vi "Create FIFO FGV Queues.vi"(8 "error in (no error)":errorcluster) -> (0 "error out":errorcluster, 4 "BC FIFO Idx Qs":T1)   [LabVIEW 2011, in "AIT 1553 Custom Device.lvlib"]
uses:
  AIT 1553 Custom Device.lvlib
  RT Controls/FIFO Idx Qs.ctl
panel:
  out "FIFO Idx Qs":T1
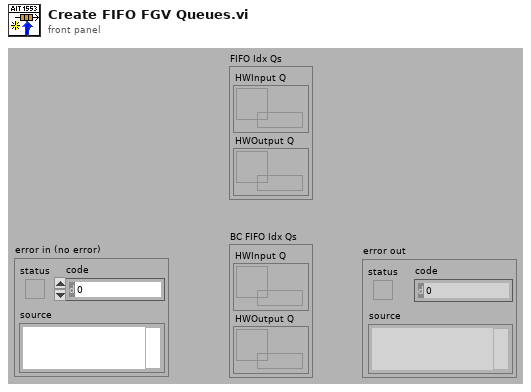
[diagram p1: front panel]
types:
  T1 = typedef "AIT 1553 Custom Device.lvlib/FIFO Idx Qs.ctl" = cluster{"HWInput Q":refnum<queue>, "HWOutput Q":refnum<queue>}
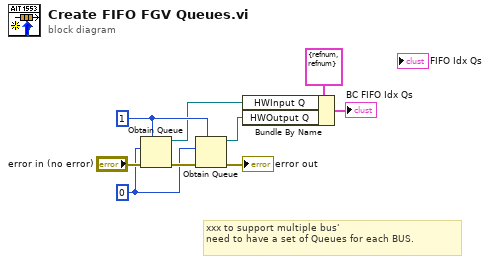
[diagram p0: block diagram]
diagram:
  w5 = 1 ("max queue size (-1, unlimited)")
  w6 = 0
  # "xxx to support multiple bus'\nneed to have a set of Queues for each BUS."
  n1 = Obtain Queue(max queue size (-1, unlimited)=w5, element data type=w6, error in (no error)="error in (no error)") -> (queue out=w3:refnum<queue>, error out=w8:errorcluster)  [unwired: 2 in, 1 out]
  n2 = Obtain Queue(max queue size (-1, unlimited)=w5, element data type=w6, error in (no error)=w8) -> (queue out=w2:refnum<queue>, error out=→"error out":errorcluster)  [unwired: 2 in, 1 out]
  n3 = Bundle By Name(cluster=T1 {"HWInput Q"=refnum, "HWOutput Q"=refnum} ("FIFO Idx Qs"), "HWInput Q"=w3, "HWOutput Q"=w2) -> (→"BC FIFO Idx Qs":T1)
